vi "matlabview.vi"(8 "Dist":dbl) -> (0 "Theta_graden":dbl)   [LabVIEW 2021]
panel:
  out "error out":errorcluster
  in  "error in (no error)":errorcluster
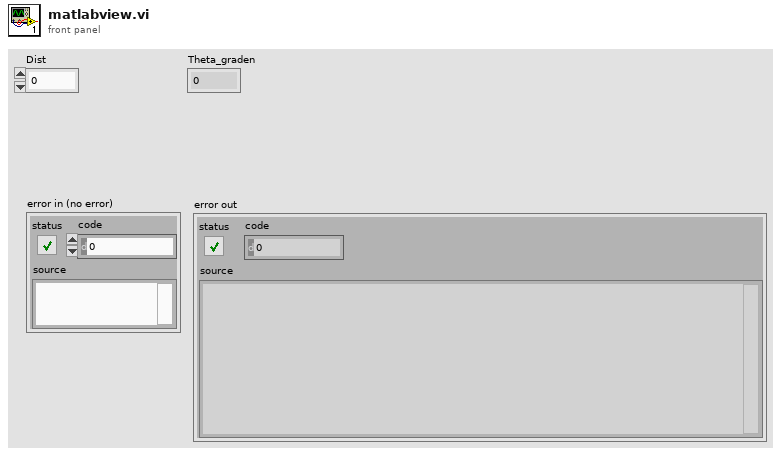
[diagram p1: front panel]
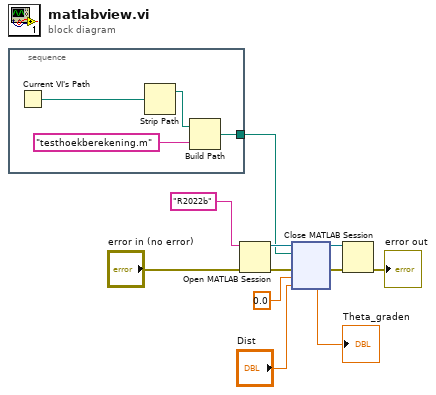
[diagram p0: block diagram]
diagram:
  n1 = stacked-sequence {
    tunnel: [w15] -> w1
    frame #0 {
      n2 = Current VI's Path() -> (path=w12:path)
      n3 = Strip Path(path=w12) -> (stripped path=w13:path)  [unwired: 1 out]
      n4 = Build Path(base path=w13, name or relative path="testhoekberekening.m") -> (appended path=w15:path)
    }
  }
  n5 = Open MATLAB Session(0:"R2022b" ("release name"), 3:"error in (no error)") -> (8:w11:refnum<k37>, 11:w6:errorcluster)
  n6 = node(w11, w1, w6, 0.0, "Dist") -> (w10:refnum<k37>, w5:errorcluster, →"Theta_graden":dbl)  [unwired: 2 in, 2 out]
  n7 = Close MATLAB Session(0:w10, 3:w5) -> (11:→"error out":errorcluster)
